vi "HFRR ADV v028 new software.vi"() -> ()   [LabVIEW 2025] (continued)
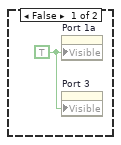
[diagram p3: hidden frame]
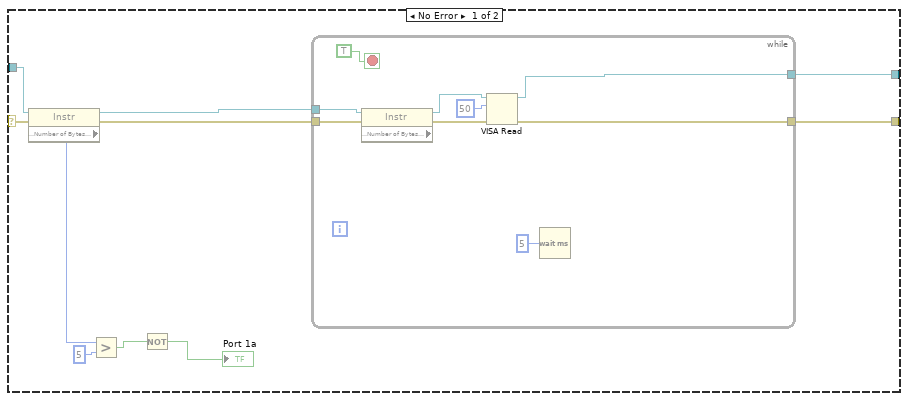
[diagram p4: hidden frame]
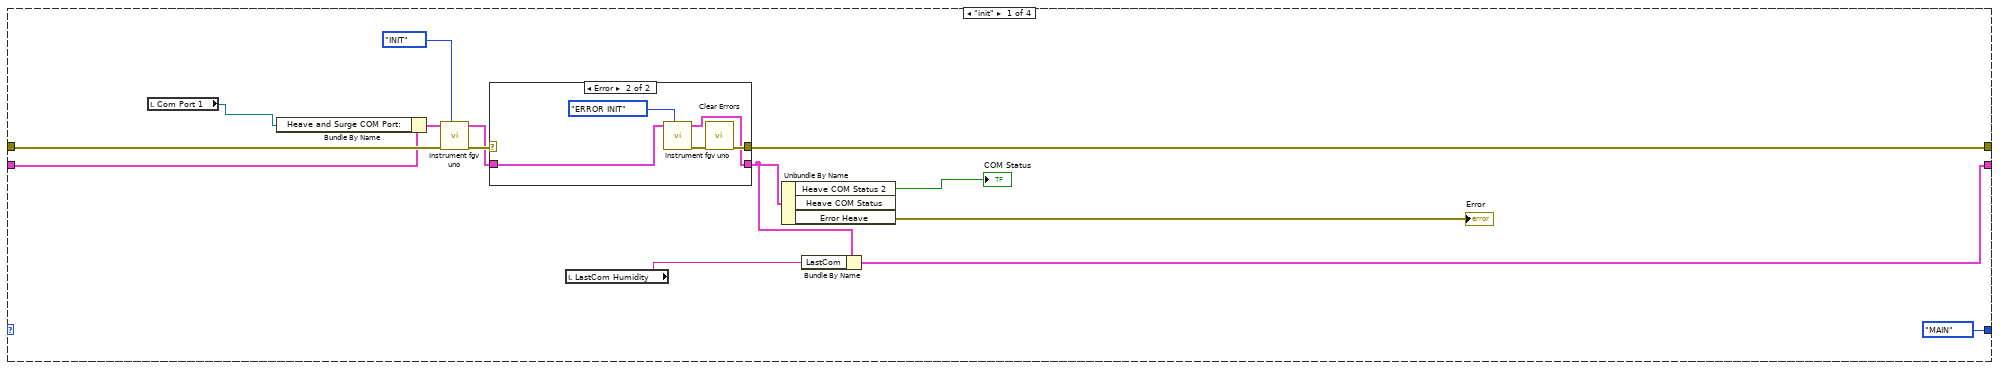
[diagram p6: hidden frame]
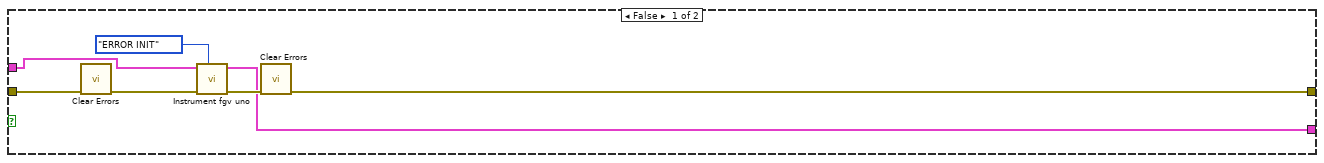
[diagram p8: hidden frame]
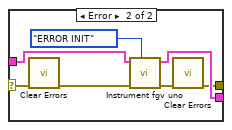
[diagram p10: hidden frame]
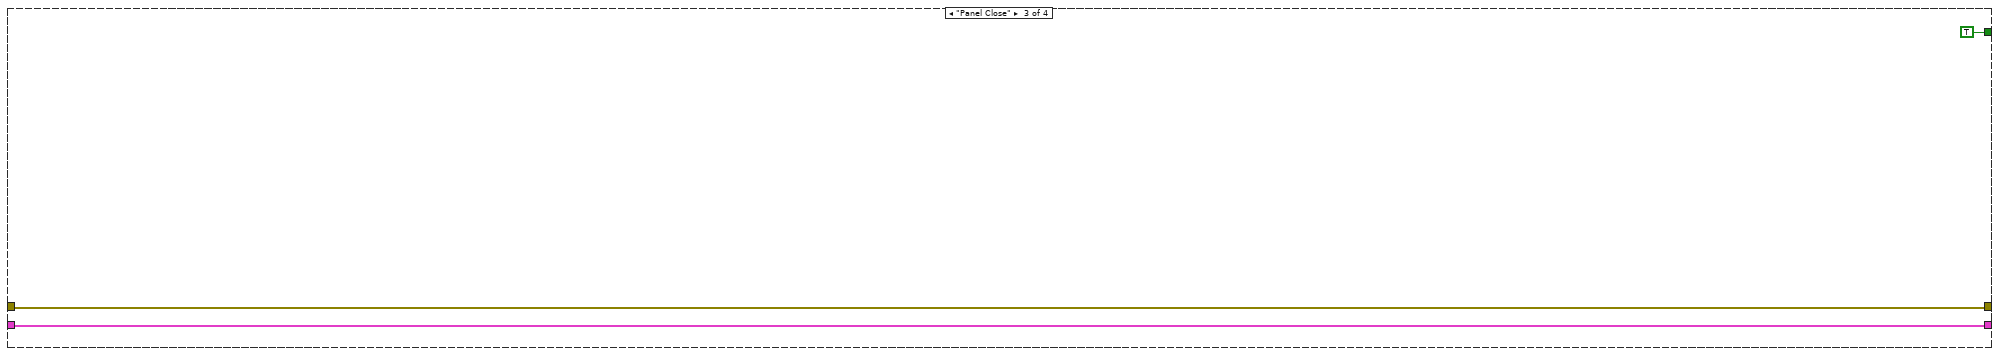
[diagram p12: hidden frame]
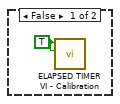
[diagram p16: hidden frame]
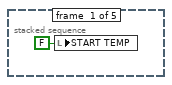
[diagram p18: hidden frame]
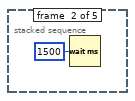
[diagram p19: hidden frame]
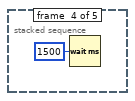
[diagram p20: hidden frame]
              tunnel: [w4454 w4456] -> w4429
              frame False {
              }
              frame True {
                n3362 = Not(x=w4462) -> (.not. x?=w4458:bool)
                n3363 = local write "Write S"(w4458) -> ()
                n3364 = call "Instrument fgv.vi"("Enum"=T29."MANUAL WRITE", "error in (no error) 2"=w4461, "INPUT"=w4457) -> ("error"=w4460:errorcluster, "output"=w4456:T18)  [unwired: 6 in, 1 out]
              }
            }
            n3365 = Array Size(array="Write UNO") -> (size(s)=w4427:i32)
            n3366 = Greater Than 0?(x=w4427) -> (x > 0?=w4426:bool)
            n3367 = call "Instrument fgv.vi"("Enum"=T29."WRITE", "error in (no error) 2"=w4430, "WriteCC1"="Write UNO", "INPUT"=w4429) -> ("error"=w4438:errorcluster, "WriteCC1 2"=w4428:string[], "output"=w4437:T18)  [unwired: 5 in]
            n3368 = case shown="True" w4426 {
              tunnel: w4428 -> [_ w4444]
              frame False {
              }
              frame True {
                n3369 = local write "Write UNO"(w4444) -> ()
              }
            }
            n3370 = case shown="Error" w4438 {
              selector: w4438 -> [w4445 w4448]
              tunnel: w4437 -> [w4446 w4453]
              tunnel: [w4446 w4452] -> w4435
              tunnel: [w4445 w4450] -> w4436
              frame No Error {
              }
              frame Error {
                n3371 = call <vilib>:"Clear Errors.vi"("error in (no error)"=w4448) -> ("error out"=w4447:errorcluster)  [unwired: 5 in, 1 out]
                n3372 = call "Instrument fgv.vi"("Enum"=T29."ERROR INIT", "error in (no error) 2"=w4447, "INPUT"=w4453) -> ("error"=w4451:errorcluster, "output"=w4452:T18)  [unwired: 6 in, 1 out]
                n3373 = call <vilib>:"Clear Errors.vi"("error in (no error)"=w4451) -> ("error out"=w4450:errorcluster)  [unwired: 5 in, 1 out]
              }
            }
            n3374 = Unbundle By Name(w4435) -> ("LastCom"=→"LastCom UNO":string, "Read Heave and Surge"=→"Read UNO":string)
          }
        }
        n3375 = Unbundle By Name(w4411) -> ("Heave COM Status 2"=w4412:bool, "Heave COM Status"=w4400:bool, "Error Heave"=w4398:errorcluster, "Bytes at Heave Port"=→"Bytes at Humidity Port":dbl)
        n3376 = Unbundle By Name(w4398) -> ()  [unwired: 1 out]
        n3377 = Not(x=w4400) -> (.not. x?=w4409:bool)
        n3378 = Not(x=w4412) -> (.not. x?=w4399:bool)
        n3379 = local write "Instrument Status"(w4409) -> ()
        n3380 = local write "Error  2"(w4398) -> ()
        n3381 = local write "Port 1a"(w4400) -> ()
        n3382 = local read "Quit"() -> (w4402:bool)
        n3383 = local write "COM Status"(w4399) -> ()
        n3384 = Select(t=enum16{"init", "MAIN", "Panel Close"}."Panel Close", s=w4402, f=enum16{"init", "MAIN", "Panel Close"}."MAIN") -> (s? t:f=w4401:enum16{"init", "MAIN", "Panel Close"})
      }
      frame "Panel Close" {
      }
      frame Default {
      }
    }
  }
  n3385 = while {
    stop <- w4493 stop-if-true
    n3386 = local read "Read HUMIDITY"() -> (w4468:string)
    n3387 = call <vilib>:"High Resolution Polling Wait.vi"("seconds to wait"=0.05) -> ()  [unwired: 10 in, 1 out]
    n3388 = Spreadsheet String To Array(delimiter (Tab)=",", format string="", spreadsheet string=w4468, array type (2D Dbl)=string[] []) -> (array=w4488:string[])
    n3389 = for {
      tunnel: w4488 -> [w4498] mode=indexing
      tunnel: string[] ["STATE;", "SET;", "RH;", "T;", "AMB_RH;", "AMB_T;", "PUMP;", "FAN_IN;", "FAN_OUT;", "DEHUM;", "CURRENT;", "STALL;"] -> [w4497] mode=indexing
      tunnel: [w4496] -> w4487 mode=indexing
      n3390 = Match Pattern(string=w4498, regular expression=w4497) -> (after substring=w4496:string)  [unwired: 1 in, 3 out]
    }
    n3391 = Index Array(array=w4487) -> (element #1=→"STATE :":string, element #2=→"SET :":string, element #3=w4476:string, element #4=→"T :":string, element #5=w4474:string, element #6=→"AMB_T :":string, element #7=→"PUMP :":string, element #8=→"FAN_IN :":string, element #9=→"FAN_OUT :":string, element #10=→"DEHUM :":string, element #11=→"CURRENT :":string, element #12=→"STALL :":string)  [unwired: 12 in]
    "RH :" <- w4476
    "AMB_RH :" <- w4474
    n3392 = Fract/Exp String To Number(string=w4476) -> (number=w4469:dbl)  [unwired: 3 in, 1 out]
    n3393 = Fract/Exp String To Number(string=w4474) -> (number=w4473:dbl)  [unwired: 3 in, 1 out]
    n3394 = local write "Ambient Humidity :"(w4473) -> ()
    n3395 = Equal?(x=w4469, y=0.0) -> (x = y?=w4471:bool)
    n3396 = case shown="True" w4471 {
      tunnel: [w4494 w4495] -> w4470
      tunnel: w4469 -> [w4494 _]
      frame False {
        (unwired) 0.0
        "Humidity temp" <- w4494
      }
      frame True {
        n3397 = local read "Humidity temp"() -> (w4495:dbl)
      }
    }
    "RH Numeric:" <- w4470
    n3398 = local read "Quit"() -> (w4493:bool)
  }
